vi "Read Elevator Position.vi"(8 "error in (no error)":errorcluster, 11 "Sim Sensor Interface Actor in":refnum<class "Sim Sensor Interface Actor.lvclass">) -> (0 "error out":errorcluster, 2 "Elevator Position":refnum<vi>, 3 "Sim Sensor Interface Actor out":refnum<class "Sim Sensor Interface Actor.lvclass">)   [LabVIEW 2022 SP3, in "Sim Sensor Interface Actor.lvlib" / "Sim Sensor Interface Actor.lvclass"]
uses:
  Sim Sensor Interface Actor.lvclass
  Sim Sensor Interface Actor.lvclass/Sim Sensor Interface Actor.ctl
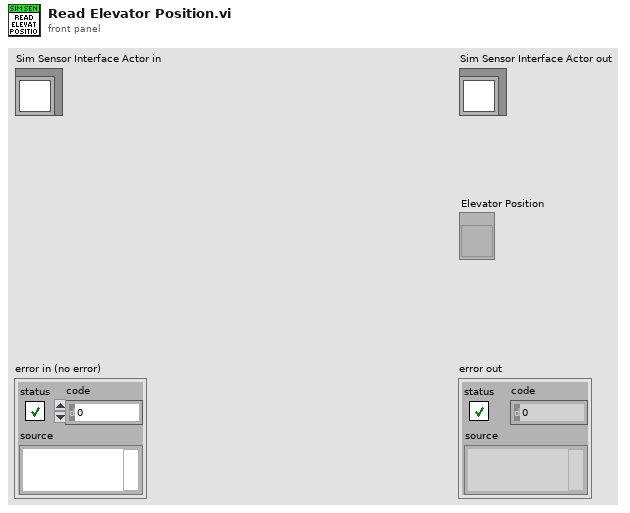
[diagram p1: front panel]
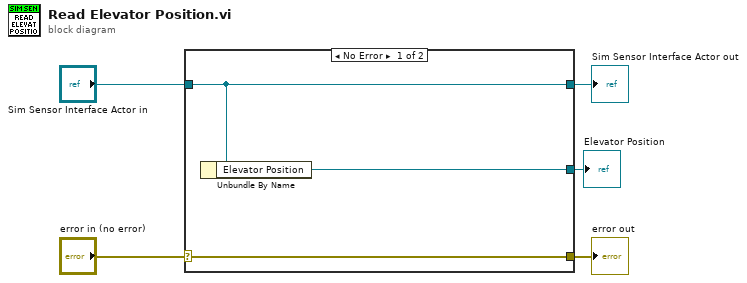
[diagram p0: block diagram]
diagram:
  n1 = case shown="No Error" "error in (no error)" {
    selector: "error in (no error)" -> [w8 w9]
    tunnel: [w8 w9] -> w4
    tunnel: [w7 w10] -> w2
    tunnel: "Sim Sensor Interface Actor in" -> [w7 w10]
    tunnel: [w6 _] -> w1
    frame No Error {
      n2 = Unbundle By Name(w7) -> ("Elevator Position"=w6:refnum<vi>)
    }
    frame Error {
    }
  }
  "error out" <- w4
  "Sim Sensor Interface Actor out" <- w2
  "Elevator Position" <- w1
